vi "PM5000_THD_demo.vi"(2 "error in (no error)":errorcluster) -> (0 "error out":errorcluster, 1 "THD_cluster":T1)   [LabVIEW 2018]
uses:
  Controls/THD_cluster.ctl
panel:
  in  "Variacion":sgl=5.0
  in  "THD":sgl=10.0
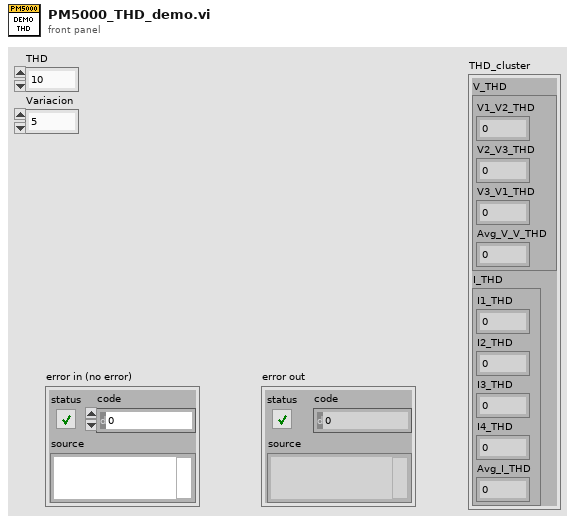
[diagram p1: front panel]
types:
  T1 = typedef "THD_cluster.ctl" = cluster{"V_THD":cluster{"V1_V2_THD":sgl, "V2_V3_THD":sgl, "V3_V1_THD":sgl, "Avg_V_V_THD":sgl}, "I_THD":cluster{"I1_THD":sgl, "I2_THD":sgl, "I3_THD":sgl, "I4_THD":sgl, "Avg_I_THD":sgl}}
  T2 = cluster{"I1_THD":sgl, "I2_THD":sgl, "I3_THD":sgl, "I4_THD":sgl, "Avg_I_THD":sgl}
  T3 = cluster{"V1_V2_THD":sgl, "V2_V3_THD":sgl, "V3_V1_THD":sgl, "Avg_V_V_THD":sgl}
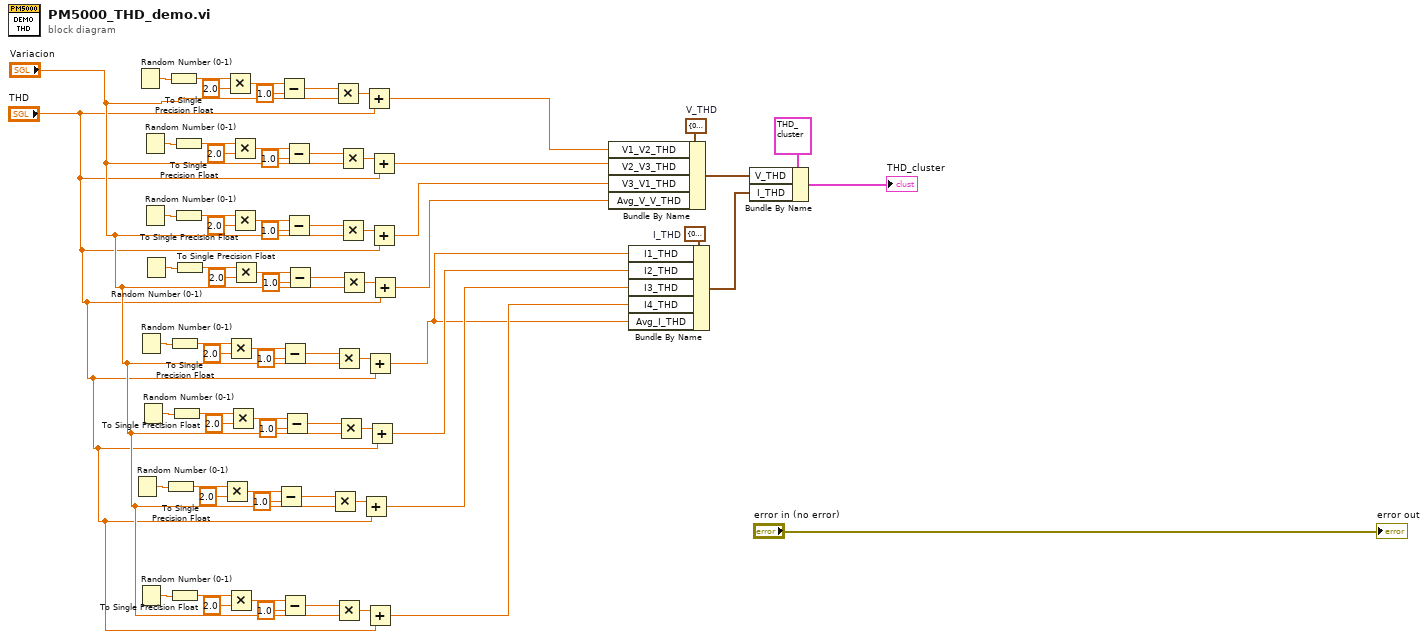
[diagram p0: block diagram]
diagram:
  w71 = T2 {"I1_THD"=0.0, "I2_THD"=0.0, "I3_THD"=0.0, "I4_THD"=0.0, "Avg_I_THD"=0.0}  # I_THD
  w72 = T3 {"V1_V2_THD"=0.0, "V2_V3_THD"=0.0, "V3_V1_THD"=0.0, "Avg_V_V_THD"=0.0}  # V_THD
  n1 = Random Number (0-1)() -> (number: 0 to 1=w21:dbl)
  n2 = Random Number (0-1)() -> (number: 0 to 1=w63:dbl)
  n3 = Random Number (0-1)() -> (number: 0 to 1=w35:dbl)
  n4 = Random Number (0-1)() -> (number: 0 to 1=w14:dbl)
  n5 = Random Number (0-1)() -> (number: 0 to 1=w28:dbl)
  n6 = Random Number (0-1)() -> (number: 0 to 1=w56:dbl)
  n7 = Random Number (0-1)() -> (number: 0 to 1=w49:dbl)
  n8 = Random Number (0-1)() -> (number: 0 to 1=w42:dbl)
  n9 = To Single Precision Float(number=w21) -> (single precision float=w20:sgl)
  n10 = To Single Precision Float(number=w63) -> (single precision float=w62:sgl)
  n11 = To Single Precision Float(number=w35) -> (single precision float=w34:sgl)
  n12 = To Single Precision Float(number=w14) -> (single precision float=w15:sgl)
  n13 = To Single Precision Float(number=w28) -> (single precision float=w29:sgl)
  n14 = To Single Precision Float(number=w56) -> (single precision float=w57:sgl)
  n15 = To Single Precision Float(number=w49) -> (single precision float=w48:sgl)
  n16 = To Single Precision Float(number=w42) -> (single precision float=w43:sgl)
  n17 = Multiply(x=w20, y=sgl 2.0) -> (x*y=w23:sgl)
  n18 = Multiply(x=w62, y=sgl 2.0) -> (x*y=w65:sgl)
  n19 = Multiply(x=w34, y=sgl 2.0) -> (x*y=w37:sgl)
  n20 = Multiply(x=w15, y=sgl 2.0) -> (x*y=w12:sgl)
  n21 = Multiply(x=w29, y=sgl 2.0) -> (x*y=w26:sgl)
  n22 = Multiply(x=w57, y=sgl 2.0) -> (x*y=w54:sgl)
  n23 = Multiply(x=w48, y=sgl 2.0) -> (x*y=w51:sgl)
  n24 = Multiply(x=w43, y=sgl 2.0) -> (x*y=w40:sgl)
  n25 = Subtract(x=w23, y=sgl 1.0) -> (x-y=w19:sgl)
  n26 = Subtract(x=w65, y=sgl 1.0) -> (x-y=w61:sgl)
  n27 = Subtract(x=w37, y=sgl 1.0) -> (x-y=w33:sgl)
  n28 = Subtract(x=w12, y=sgl 1.0) -> (x-y=w16:sgl)
  n29 = Subtract(x=w26, y=sgl 1.0) -> (x-y=w30:sgl)
  n30 = Subtract(x=w54, y=sgl 1.0) -> (x-y=w58:sgl)
  n31 = Subtract(x=w51, y=sgl 1.0) -> (x-y=w47:sgl)
  n32 = Subtract(x=w40, y=sgl 1.0) -> (x-y=w44:sgl)
  n33 = Multiply(x=w19, y="Variacion") -> (x*y=w18:sgl)
  n34 = Multiply(x=w61, y="Variacion") -> (x*y=w60:sgl)
  n35 = Multiply(x=w33, y="Variacion") -> (x*y=w32:sgl)
  n36 = Multiply(x=w16, y="Variacion") -> (x*y=w17:sgl)
  n37 = Multiply(x=w30, y="Variacion") -> (x*y=w31:sgl)
  n38 = Multiply(x=w58, y="Variacion") -> (x*y=w59:sgl)
  n39 = Multiply(x=w47, y="Variacion") -> (x*y=w46:sgl)
  n40 = Multiply(x=w44, y="Variacion") -> (x*y=w45:sgl)
  n41 = Add(x=w18, y="THD") -> (x+y=w3:sgl)
  n42 = Add(x=w60, y="THD") -> (x+y=w8:sgl)
  n43 = Add(x=w32, y="THD") -> (x+y=w1:sgl)
  n44 = Add(x=w17, y="THD") -> (x+y=w2:sgl)
  n45 = Add(x=w31, y="THD") -> (x+y=w4:sgl)
  n46 = Add(x=w59, y="THD") -> (x+y=w7:sgl)
  n47 = Add(x=w46, y="THD") -> (x+y=w6:sgl)
  n48 = Add(x=w45, y="THD") -> (x+y=w5:sgl)
  n49 = Bundle By Name(cluster=w72, "V1_V2_THD"=w8, "V2_V3_THD"=w7, "V3_V1_THD"=w6, "Avg_V_V_THD"=w5) -> (w69:T3)
  n50 = Bundle By Name(cluster=w71, "I1_THD"=w1, "I2_THD"=w4, "I3_THD"=w3, "I4_THD"=w2, "Avg_I_THD"=w1) -> (w68:T2)
  n51 = Bundle By Name(cluster=T1 {"V_THD"={"V1_V2_THD"=0.0, "V2_V3_THD"=0.0, "V3_V1_THD"=0.0, "Avg_V_V_THD"=0.0}, "I_THD"={"I1_THD"=0.0, "I2_THD"=0.0, "I3_THD"=0.0, "I4_THD"=0.0, "Avg_I_THD"=0.0}} ("THD_cluster"), "V_THD"=w69, "I_THD"=w68) -> (→"THD_cluster":T1)
  "error out" <- "error in (no error)"
